vi "analise_instabilidade.vi"() -> ()   [LabVIEW 2013]
uses:
  <vilib>/Instr/_visa.llb/VISA Configure Serial Port (Instr).vi
panel:
  out "n":i32[](array[numeric])
  out "output_data 2":u8[](array[numeric])
  in  "offset":i32
  out "offset_value":i32[](array[numeric])
  in  "Controle":i32=12
  in  "atual":i32
  out "output_data":u8[](array[numeric])
  out "atualOut":i32[](array[numeric])
  in  "baud rate":u32=9600
  in  "t2":dbl
  in  "t1":dbl
  in  "stop":bool
  out "time dt(ms)":dbl
  in  "serial_port":refnum<visa-resource-name> caption="Porta Serial"
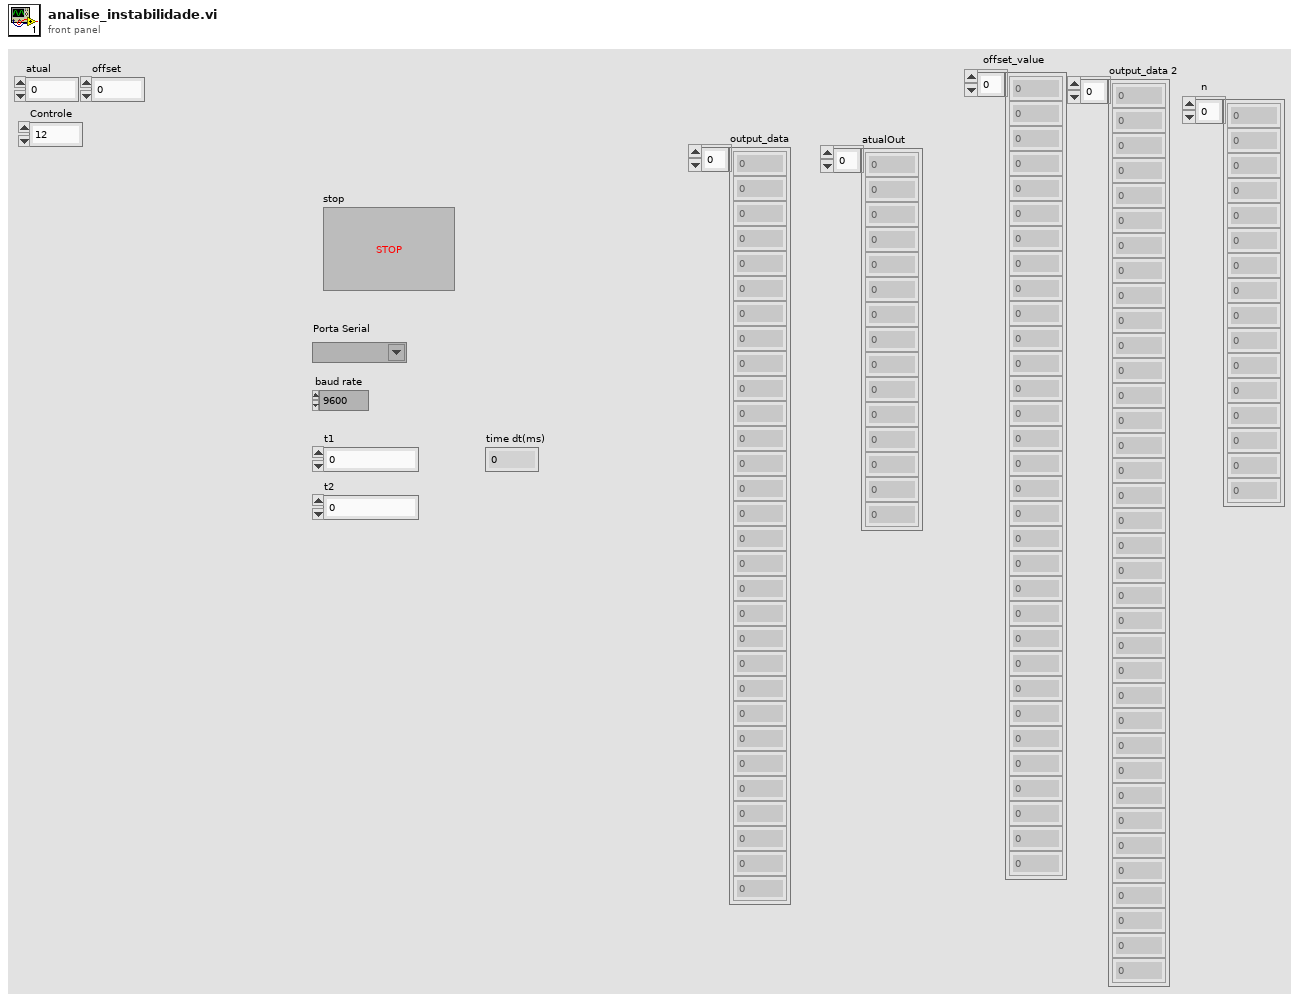
[diagram p1: front panel]
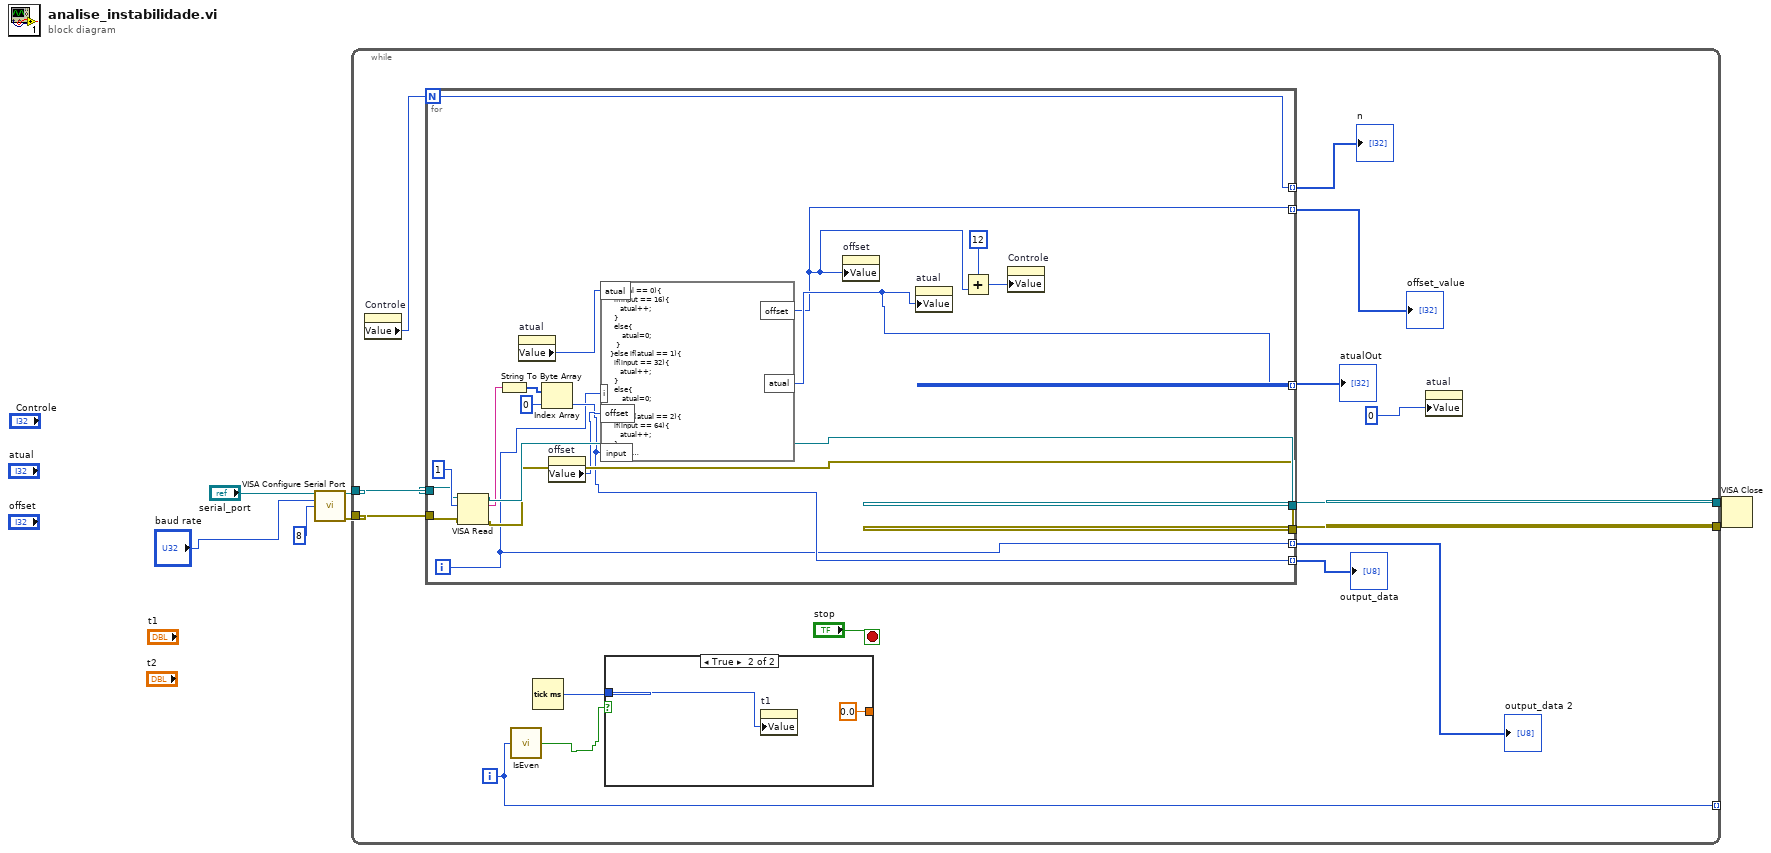
[diagram p0: block diagram]
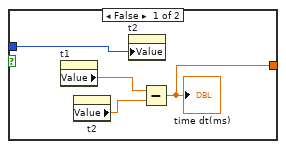
[diagram p2: hidden frame]
diagram:
  n1 = call-poly "VISA Configure Serial Port"("VISA resource name"="serial_port", "baud rate (9600)"="baud rate", "data bits (8)"=u16 8) -> ("VISA resource name out"=w5:refnum<visa-resource-name>, "error out"=w4:errorcluster)  [unwired: 11 in]
  n2 = while {
    tunnel: w5 -> [w18]
    tunnel: w4 -> [w19]
    tunnel: [w16] -> w3
    tunnel: [w17] -> w2
    tunnel: [w15] -> _ mode=indexing
    i -> [w15]
    stop <- "stop" stop-if-true
    n3 = property on="Controle" class="DigNum (strict)"() -> ("Value"=w12:i32)  [unwired: 2 in, 2 out]
    n4 = for {
      N: w12 -> [w25]
      tunnel: w19 -> [w38]
      tunnel: w18 -> [w37]
      tunnel: [w36] -> w17
      tunnel: [w35] -> w16
      tunnel: [w26] -> w14 mode=indexing
      tunnel: [w29] -> w13 mode=indexing
      tunnel: [w23] -> w11 mode=indexing
      tunnel: [w27] -> w10 mode=indexing
      tunnel: [w25] -> w9 mode=indexing
      i -> [w27]
      n5 = VISA Read(VISA resource name=w37, byte count=1, error in (no error)=w38) -> (VISA resource name out=w36:refnum<visa-resource-name>, read buffer=w34:string, error out=w35:errorcluster)  [unwired: 1 out]
      n6 = String To Byte Array(string=w34) -> (unsigned byte array=w32:u8[])
      n7 = property on="atual" class="DigNum (strict)"() -> ("Value"=w31:i32)  [unwired: 2 in, 2 out]
      n8 = Index Array(array=w32, index=0) -> (element=w29:u8)
      n9 = property on="offset" class="DigNum (strict)"() -> ("Value"=w30:i32)  [unwired: 2 in, 2 out]
      n10 = formula code="if(atual == 0){\n  if(input == 16){\n     atual++;\n  }\n  else{\n      atual=0;\n   }\n}else if(atual == 1){\n  if(input == 32){\n     atual++;\n  }\n  else{\n      atual=0;\n   }\n}else if(atual == 2){\n  if(input == 64){\n     atual++;\n  }\n  else{\n      atual=0;\n   }\n}else if(atual == 3){\n\n  if(input == 128){\n     atual++;\n  }\n  else{\n      atual=0;\n   }\n}\nelse{\n if(atual == 4)\n    offset = i-4; \n\n  atual++;\n  if(atual >= 12)\n     atual = 0 ;\n}"("atual"=w31, "input"=w29, "i"=w27, "offset"=w30) -> ("atual"=w26:i32, "offset"=w23:i32)
      n11 = property on="offset" class="DigNum (strict)"("Value"=w23) -> ()  [unwired: 2 in, 2 out]
      n12 = property on="atual" class="DigNum (strict)"("Value"=w26) -> ()  [unwired: 2 in, 2 out]
      n13 = Add(x=u16 12 ("data bits (8)"), y=w23) -> (x+y=w28:i32)
      n14 = property on="Controle" class="DigNum (strict)"("Value"=w28) -> ()  [unwired: 2 in, 2 out]
    }
    "atualOut" <- w14
    "output_data" <- w13
    "offset_value" <- w11
    "output_data 2" <- w10
    "n" <- w9
    n15 = call "IsEven.vi"("Numeric"=w15) -> ("Boolean"=w20:bool)
    n16 = Tick Count (ms)() -> (millisecond timer value=w21:u32)
    n17 = case shown="True" w20 {
      tunnel: w21 -> [w43 w45]
      tunnel: [w40 0.0] -> _
      frame False {
        n18 = property on="t1" class="DigNum (strict)"() -> ("Value"=w42:dbl)  [unwired: 2 in, 2 out]
        n19 = property on="t2" class="DigNum (strict)"() -> ("Value"=w41:dbl)  [unwired: 2 in, 2 out]
        n20 = property on="t2" class="DigNum (strict)"("Value"=w43) -> ()  [unwired: 2 in, 2 out]
        n21 = Subtract(x=w42, y=w41) -> (x-y=w40:dbl)
        "time dt(ms)" <- w40
      }
      frame True {
        n22 = property on="t1" class="DigNum (strict)"("Value"=w45) -> ()  [unwired: 2 in, 2 out]
      }
    }
    n23 = property on="atual" class="DigNum (strict)"("Value"=0) -> ()  [unwired: 2 in, 2 out]
  }
  n24 = VISA Close(VISA resource name=w2, error in (no error)=w3) -> ()  [unwired: 1 out]
